vi "apply_password.vi"() -> ()   [LabVIEW 2020]
panel:
  in  "Apply Password":bool=TRUE
  out "error out":errorcluster
  in  "Password":string="Iam$oliton"
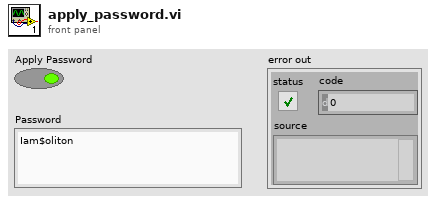
[diagram p1: front panel]
types:
  T1 = enum32{"invalid lock state", "Not Locked", "Locked (No Password)", "Password-protected"}
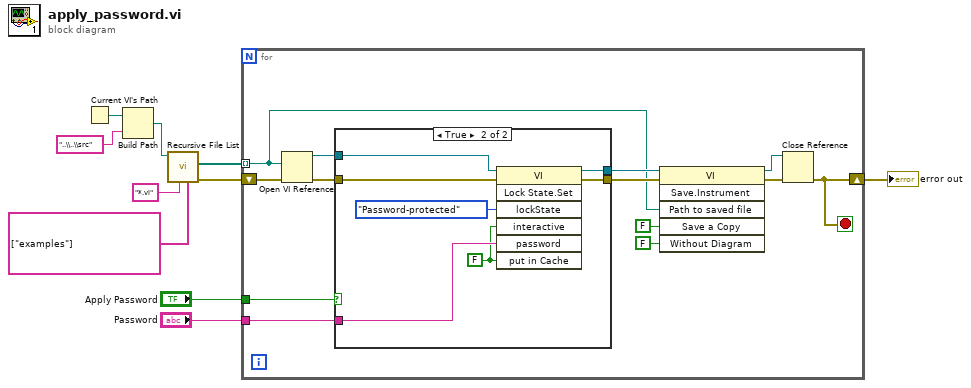
[diagram p0: block diagram]
diagram:
  n1 = Current VI's Path() -> (path=w10:path)
  n2 = Build Path(base path=w10, name or relative path="..\\..\\src") -> (appended path=w8:path)
  n3 = call <vilib>:"Recursive File List.vi"("Folders to Exclude"=string[] ["examples"], "pattern"="*.vi", "Folder Path"=w8) -> ("error out"=w1:errorcluster, "All Files in Dir"=w5:path[])  [unwired: 4 in, 3 out]
  n4 = for {
    tunnel: w5 -> [w17] mode=indexing
    tunnel: "Password" -> [w20]
    tunnel: "Apply Password" -> [w13]
    shift-right: [w12] -> w3
    shift-left: w1 -> [w23]
    stop <- w12 stop-if-true
    n5 = Open VI Reference(vi path=w17, error in (no error)=w23) -> (vi reference=w21:refnum<vi>, error out=w22:errorcluster)  [unwired: 4 in]
    n6 = case shown="True" w13 {
      tunnel: w22 -> [w25 w32]
      tunnel: w21 -> [w24 w31]
      tunnel: w20 -> [_ w29]
      tunnel: [w25 w27] -> w19
      tunnel: [w24 w26] -> w18
      frame False {
      }
      frame True {
        w28 = FALSE ("Put in Cache")
        n7 = invoke class="VI" method="Lock State.Set"(reference=w31, error in=w32, "lockState"=T1."Password-protected" ("Lock State"), "interactive"=w28, "password"=w29, "put in Cache"=w28) -> (reference out=w26:refnum<vi>, error out=w27:errorcluster)  [unwired: 1 in, 5 out]
      }
    }
    n8 = invoke class="VI" method="Save.Instrument"(reference=w18, error in=w19, "Path to saved file"=w17, "Save a Copy"=FALSE, "Without Diagram"=FALSE) -> (reference out=w14:refnum<vi>, error out=w15:errorcluster)  [unwired: 1 in, 4 out]
    n9 = Close Reference(reference=w14, error in (no error)=w15) -> (error out=w12:errorcluster)
  }
  "error out" <- w3
